vi "Create Plugin Tree Tag.vi"(7 "ItemType":T1, 8 "error in (no error)":errorcluster, 9 "Script":string[](array[string]), 10 "Name":string(combo), 11 "VISA Resource":path caption="Path") -> (0 "error out":errorcluster, 2 "Name out":string(combo) caption="Name", 3 "Tag":string)   [LabVIEW 2018]
uses:
  Controls/Plugins Tree Item Type.ctl
  Controls/Plugin Tree Tag.ctl
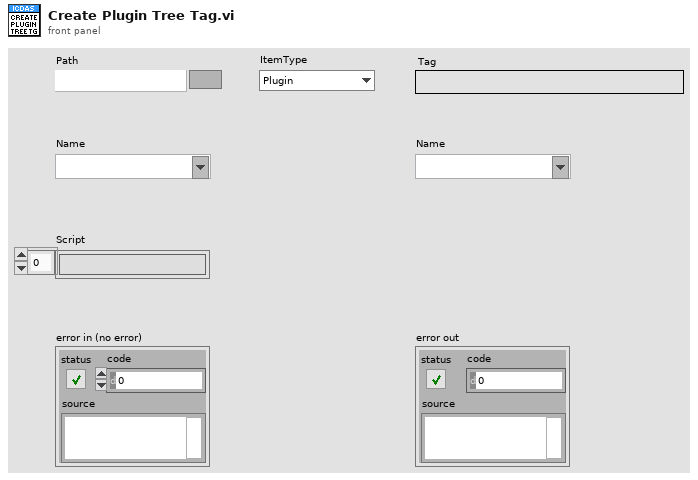
[diagram p1: front panel]
types:
  T1 = typedef "Plugins Tree Item Type.ctl" = enum16{"Plugin", "Instrument", "INI File", "INI Script"}
  T2 = typedef "Plugin Tree Tag.ctl" = cluster{"ItemType":T1, "Name":string, "Path":path, "Script":string[]}
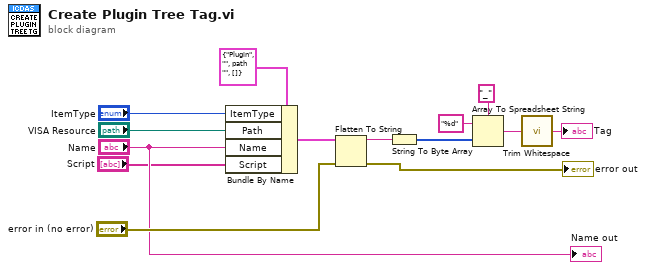
[diagram p0: block diagram]
diagram:
  n1 = Bundle By Name(cluster=T2 {"ItemType"=enum."Plugin", "Name"="", "Path"=path "", "Script"=[]} ("Test Manager Tree Tag"), "ItemType"="ItemType", "Path"="VISA Resource", "Name"="Name", "Script"="Script") -> (w13:T2)
  n2 = Flatten To String(anything=w13, error in (no error)="error in (no error)") -> (data string=w10:string, error out=→"error out":errorcluster)  [unwired: 2 in, 1 out]
  n3 = String To Byte Array(string=w10) -> (unsigned byte array=w9:u8[])
  n4 = Array To Spreadsheet String(delimiter (Tab)="_" ("format string"), array=w9, 3:"%d" ("format string")) -> (spreadsheet string=w6:string)
  n5 = call <vilib>:"Trim Whitespace.vi"("string"=w6) -> ("trimmed string"=→"Tag":string)  [unwired: 1 in]
  "Name out" <- "Name"
